vi "RSZVB Set Trace Display State.vi"(7 "Show Trace":bool=TRUE, 8 "error in (no error)":errorcluster {"code" format="%.0x"}, 9 "Single Trace Name (\"Trc1\")":string="Trc1", 10 "Trace Type (0)":i32(ring) items=["All Data Traces", "All Memory Traces", "Single Trace"], 11 "VISA session":refnum<visa-resource-name>) -> (0 "error out":errorcluster {"code" format="%.0x"}, 3 "dup VISA session":refnum<visa-resource-name>)   [LabVIEW 2011]
doc: "Displays or hides an existing trace, identified by its trace name (CALCulate<Ch>:PARameter:SDEFine <Trace_Name>), or a group of traces.\n\nRemote-control command(s):\nDISPlay[:WINDow<Wnd>]:TRACe<WndTr>:SHOW DALL | MALL | '<trace_name>', <Boolean>"
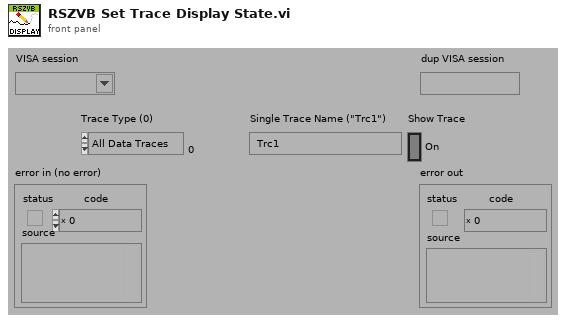
[diagram p1: front panel]
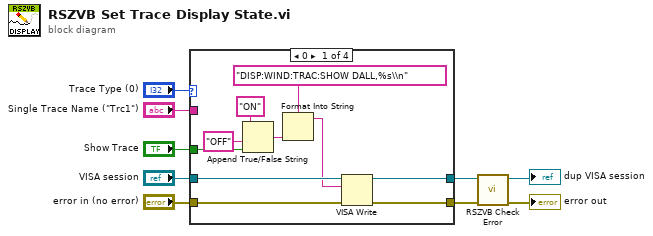
[diagram p0: block diagram]
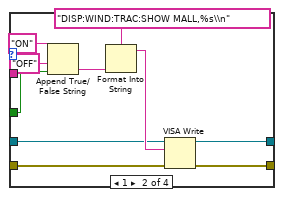
[diagram p2: hidden frame]
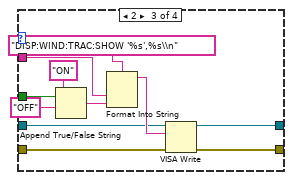
[diagram p3: hidden frame]
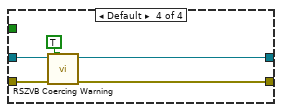
[diagram p4: hidden frame]
diagram:
  n1 = case shown="0" "Trace Type (0)" {
    tunnel: "VISA session" -> [w14 w24 w35 w44]
    tunnel: "error in (no error)" -> [w13 w23 w36 w45]
    tunnel: "Show Trace" -> [w19 w20 w32 _]
    tunnel: "Single Trace Name (\"Trc1\")" -> [_ _ w31 _]
    tunnel: [w11 w22 w33 w43] -> w4
    tunnel: [w10 w21 w34 w42] -> w3
    frame 0 {
      n2 = Append True/False String(1:w19, 2:"OFF" ("false string"), 3:"ON" ("true string")) -> (0:w15:string)  [unwired: 1 in]
      n3 = Format Into String(format string="DISP:WIND:TRAC:SHOW DALL,%s\\n", w15) -> (resulting string=w12:string)  [unwired: 2 in, 1 out]
      n4 = VISA Write(VISA resource name=w14, write buffer=w12, error in (no error)=w13) -> (VISA resource name out=w10:refnum<visa-resource-name>, error out=w11:errorcluster)  [unwired: 1 out]
    }
    frame 1 {
      n5 = Append True/False String(1:w20, 2:"OFF" ("false string"), 3:"ON" ("true string")) -> (0:w26:string)  [unwired: 1 in]
      n6 = Format Into String(format string="DISP:WIND:TRAC:SHOW MALL,%s\\n", w26) -> (resulting string=w25:string)  [unwired: 2 in, 1 out]
      n7 = VISA Write(VISA resource name=w24, write buffer=w25, error in (no error)=w23) -> (VISA resource name out=w21:refnum<visa-resource-name>, error out=w22:errorcluster)  [unwired: 1 out]
    }
    frame 2 {
      n8 = Append True/False String(1:w32, 2:"OFF" ("false string"), 3:"ON" ("true string")) -> (0:w30:string)  [unwired: 1 in]
      n9 = Format Into String(format string="DISP:WIND:TRAC:SHOW '%s',%s\\n", w31, w30) -> (resulting string=w37:string)  [unwired: 2 in, 1 out]
      n10 = VISA Write(VISA resource name=w35, write buffer=w37, error in (no error)=w36) -> (VISA resource name out=w34:refnum<visa-resource-name>, error out=w33:errorcluster)  [unwired: 1 out]
    }
    frame Default {
      n11 = call "RSZVB Coercing Warning.vi"("In Range?"=TRUE, "error in (no error)"=w45, "VISA session"=w44) -> ("error out"=w43:errorcluster, "dup VISA session"=w42:refnum<visa-resource-name>)  [unwired: 7 in]
    }
  }
  n12 = call "RSZVB Check Error.vi"("error in (no error)"=w4, "VISA session"=w3) -> ("error out"=→"error out":errorcluster, "dup VISA session"=→"dup VISA session":refnum<visa-resource-name>)  [unwired: 8 in]
